vi "Start Data Stream.vi"(8 "error in (no error)":errorcluster, 11 "Statnett C37.118 DLL in":refnum<class "Statnett C37.118 DLL.lvclass">) -> (0 "error out":errorcluster, 3 "Statnett C37.118 DLL out":refnum<class "Statnett C37.118 DLL.lvclass">)   [LabVIEW 2013, in "PMU Recorder Light.lvlib" / "Statnett C37.118 DLL.lvclass"]
uses:
  Statnett C37.118 DLL.lvclass
  Statnett C37.118 DLL.lvclass/Statnett C37.118 DLL.ctl
  c37118-dll/labview/C37118-DLL.lvlib
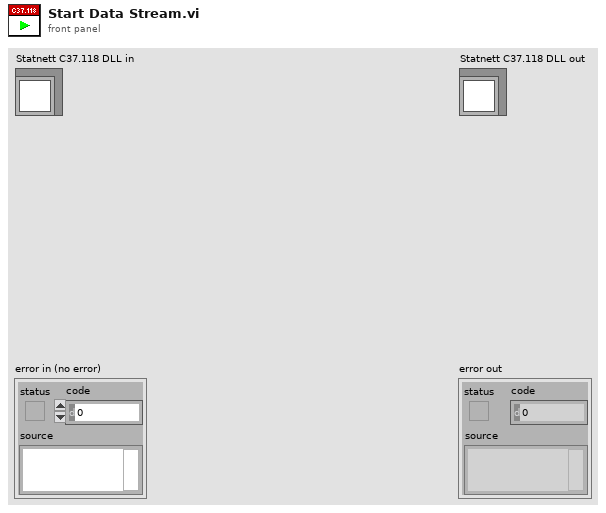
[diagram p1: front panel]
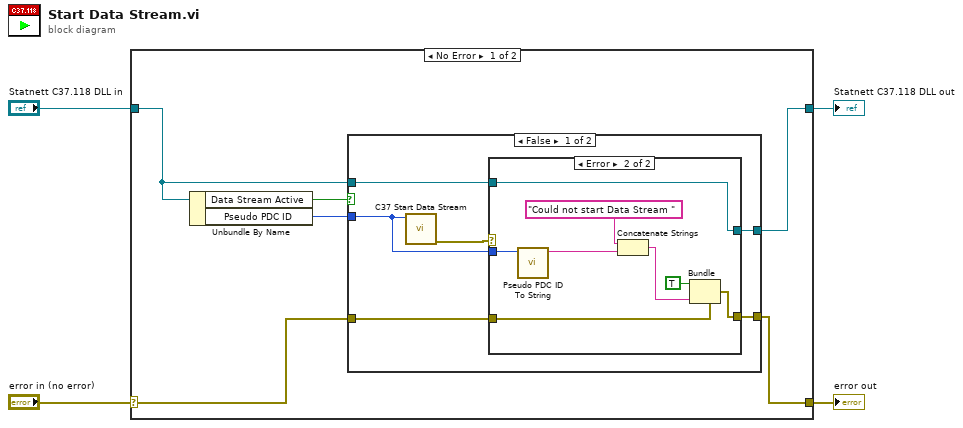
[diagram p0: block diagram]
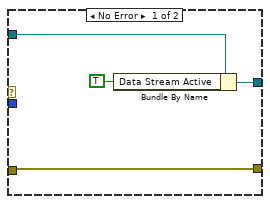
[diagram p2: hidden frame]
diagram:
  n1 = case shown="No Error" "error in (no error)" {
    selector: "error in (no error)" -> [w6 w32]
    tunnel: [w5 w32] -> w3
    tunnel: [w7 w31] -> w1
    tunnel: "Statnett C37.118 DLL in" -> [w8 w31]
    frame No Error {
      n2 = Unbundle By Name(w8) -> ("Data Stream Active"=w9:bool, "Pseudo PDC ID"=w10:i32)
      n3 = case shown="False" w9 {
        tunnel: w10 -> [w12 _]
        tunnel: w8 -> [w16 w30]
        tunnel: [w15 w30] -> w7
        tunnel: w6 -> [w14 w29]
        tunnel: [w13 w29] -> w5
        frame False {
          n4 = call "C37 Start Data Stream.vi"("Pseudo PDC ID"=w12) -> ("error out"=w11:errorcluster)  [unwired: 10 in]
          n5 = case shown="Error" w11 {
            tunnel: w16 -> [w20 w24]
            tunnel: [w18 w24] -> w15
            tunnel: w12 -> [_ w23]
            tunnel: w14 -> [w17 w22]
            tunnel: [w17 w21] -> w13
            frame No Error {
              n6 = Bundle By Name(cluster=w20, "Data Stream Active"=TRUE) -> (w18:refnum<class "Statnett C37.118 DLL.lvclass">)
            }
            frame Error {
              n7 = call "Pseudo PDC ID To String.vi"("Pseudo PDC ID"=w23) -> ("String"=w25:string)  [unwired: 10 in]
              n8 = Concatenate Strings("Could not start Data Stream " ("source"), w25) -> (w28:string)
              n9 = Bundle(cluster=w22, "status"=TRUE, "source"=w28) -> (w21:errorcluster)  [unwired: 1 in]
            }
          }
        }
        frame True {
        }
      }
    }
    frame Error {
    }
  }
  "error out" <- w3
  "Statnett C37.118 DLL out" <- w1
